vi "Go.vi"(9 "Timing Data":T1(array[cluster]), 10 "Control In":T2={"I-O.lvclass"=refnum, "Gantry"=refnum, "Dispenser"="COM1"}, 11 "Sensor Dispense in":refnum<class "Sensor Dispense.lvclass">) -> (2 "Control Out":T2={"I-O.lvclass"=refnum, "Gantry"=refnum, "Dispenser"="COM1"}, 3 "Sensor Dispense out":refnum<class "Sensor Dispense.lvclass">)   [LabVIEW 2021, in "Sensor Dispense.lvclass"]
uses:
  Sensor Dispense.lvclass
  C:/Users/hep/Documents/UCSB-CMU-GantryCode/UCSB-Gantry-HEP-main (3)/UCSB-Gantry-HEP-main/Classes/Routine/Dispense/Dispense.lvclass
  Classes/Controller/Controllers.ctl
  Classes/Controller/I-O/I-O.lvclass
  C:/Program Files (x86)/Aerotech/A3200/LabVIEW/2010/Bin/Aerotech.A3200.dll
  Program Files (x86)/Aerotech/A3200/LabVIEW/2010/Bin/Aerotech.A3200.dll
  Sensor Dispense.lvclass/Sensor Dispense.ctl
  Classes/Controller/Motion/Motion.lvclass
  Classes/Controller/Dispenser/Dispenser.lvclass
  Classes/Controller/Motion/A3200/A3200.lvclass
  Classes/Controller/Controller.lvclass
panel:
  out "error out":errorcluster
  in  "error in (no error)":errorcluster
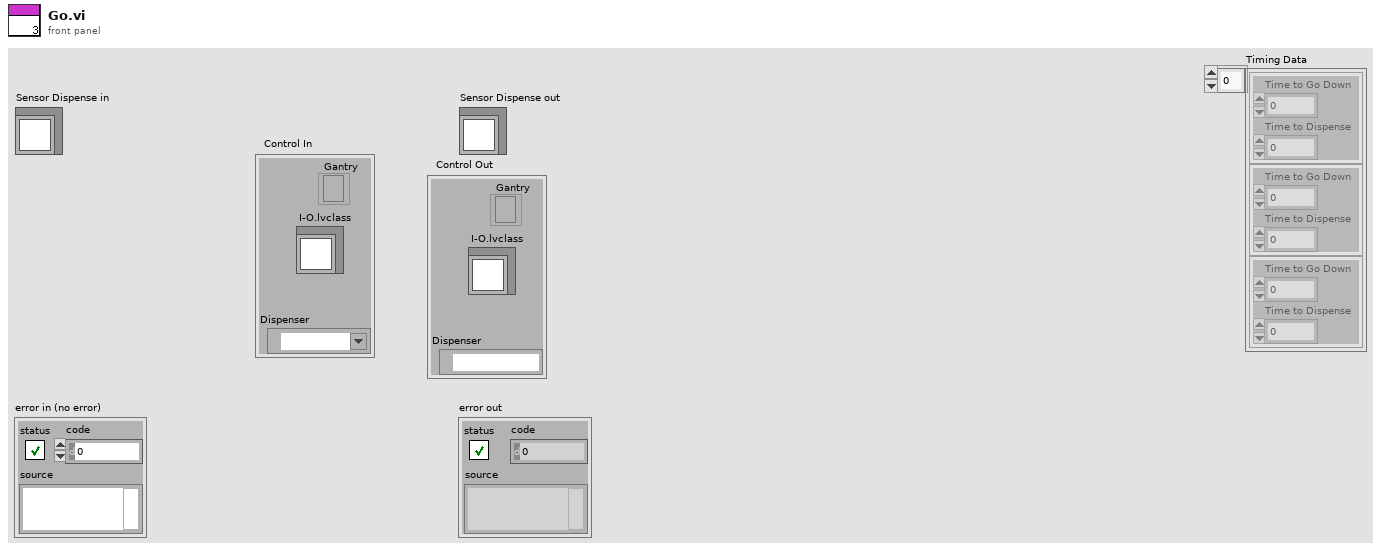
[diagram p1: front panel]
types:
  T1 = cluster{"Time to Go Down":i32, "Time to Dispense":i32}[]
  T2 = typedef "Controller.lvclass/Controllers.ctl" = cluster{"I-O.lvclass":refnum<class "I-O.lvclass">, "Gantry":refnum<k24>, "Dispenser":refnum<visa-resource-name>}
  T3 = cluster{"Endpoints":dbl[][], "Center":dbl[], "CW/CCW":dbl, "Dispense Type":enum16{"N-gon", "Square", "Arc", "Dot", "Line", "Circle"}}[]
  T4 = cluster{"Endpoints":dbl[][], "Center":dbl[], "CW/CCW":dbl, "Dispense Type":enum16{"N-gon", "Square", "Arc", "Dot", "Line", "Circle"}}
  T5 = enum16{"N-gon", "Square", "Arc", "Dot", "Line", "Circle"}
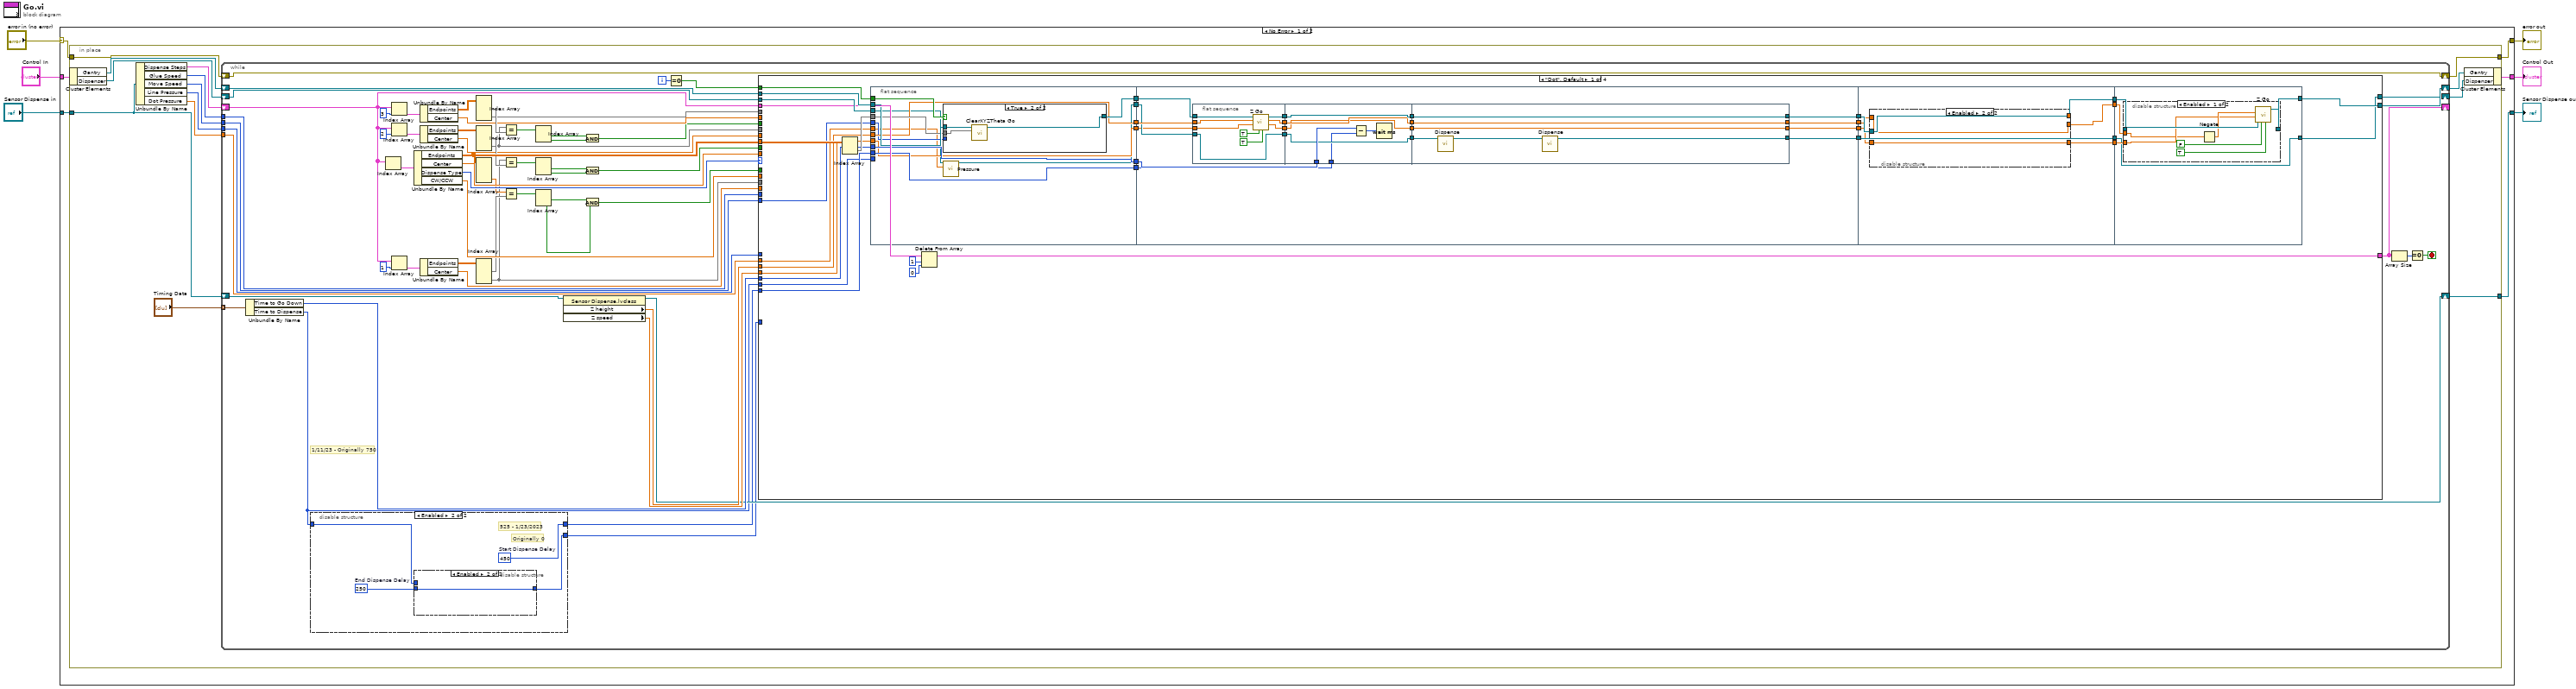
[diagram p0: block diagram]
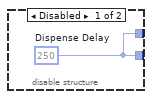
[diagram p2: hidden frame]
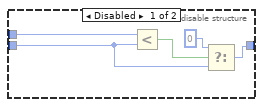
[diagram p3: hidden frame]
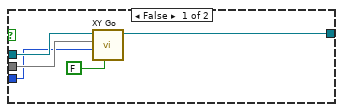
[diagram p4: hidden frame]
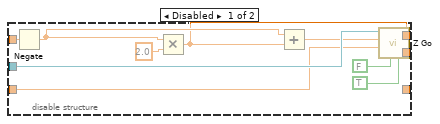
[diagram p5: hidden frame]
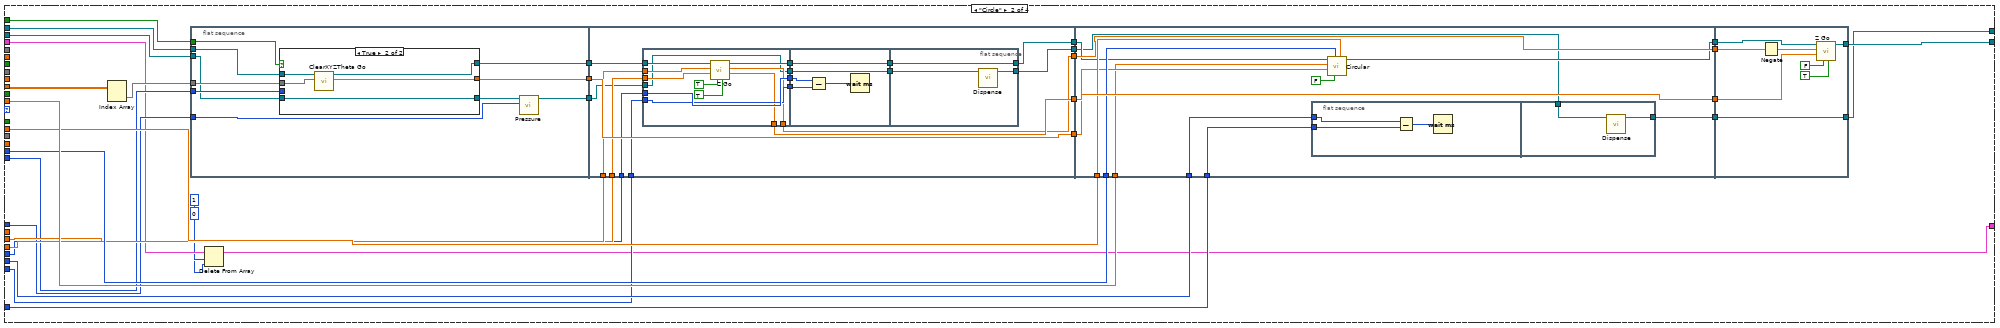
[diagram p7: hidden frame]
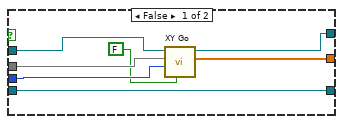
[diagram p8: hidden frame]
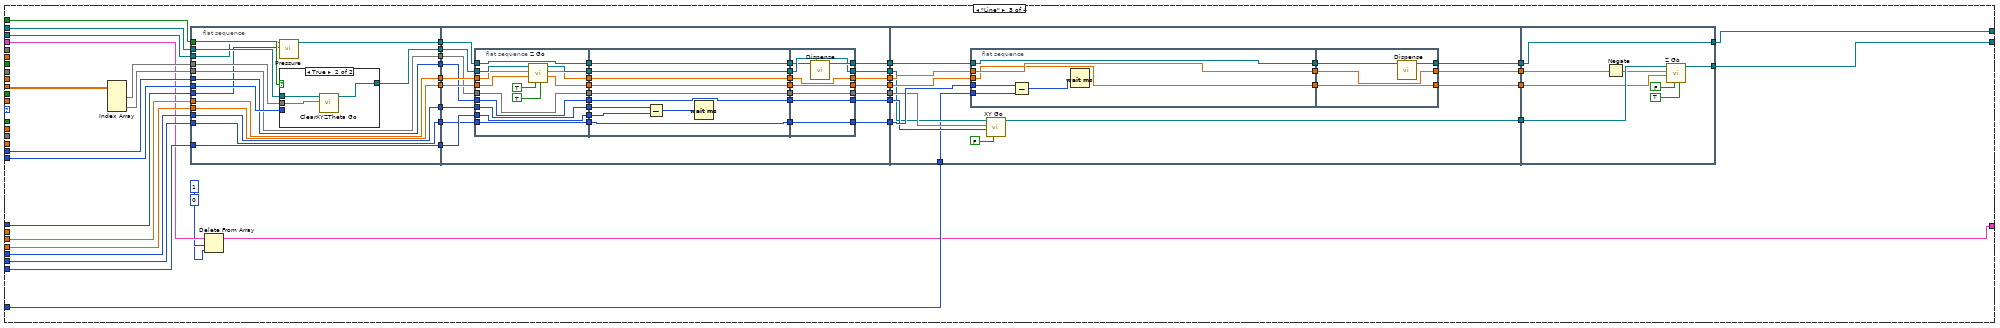
[diagram p9: hidden frame]
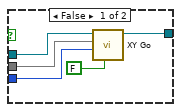
[diagram p10: hidden frame]
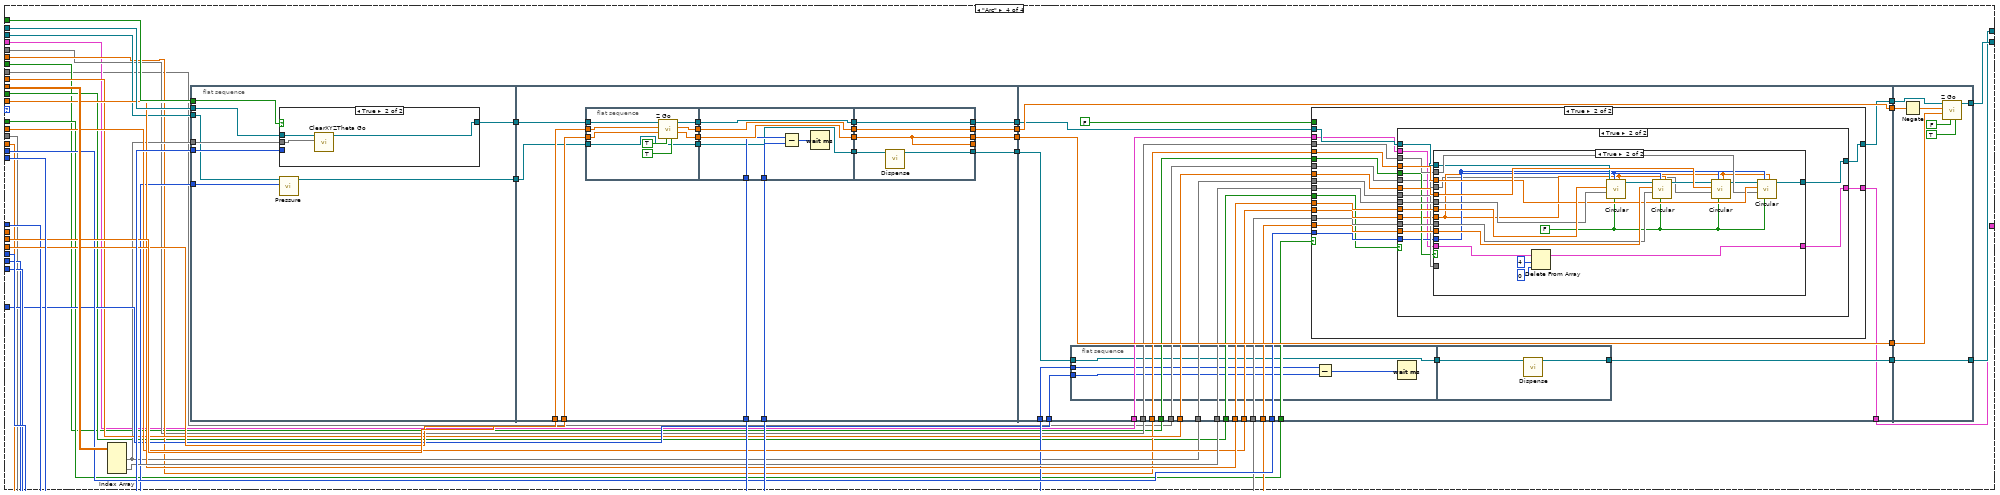
[diagram p11: hidden frame]
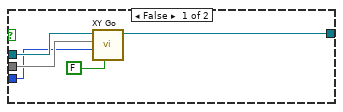
[diagram p12: hidden frame]
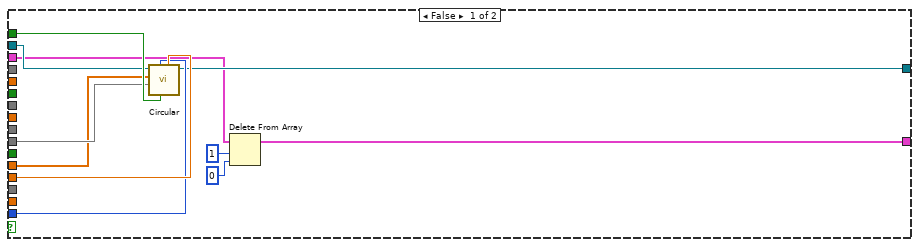
[diagram p13: hidden frame]
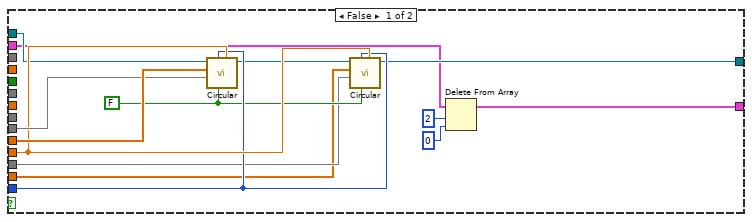
[diagram p14: hidden frame]
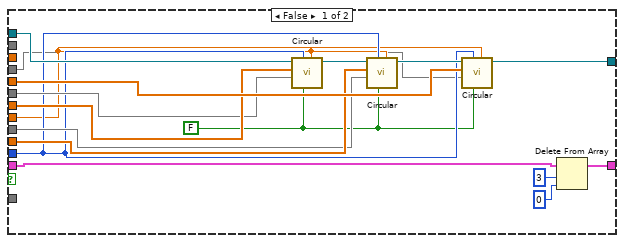
[diagram p15: hidden frame]
diagram:
  n1 = case shown="No Error" "error in (no error)" {
    selector: "error in (no error)" -> [w7 w735]
    tunnel: "Sensor Dispense in" -> [w12 w734]
    tunnel: [w11 w734] -> w5
    tunnel: "Control In" -> [w10 w733]
    tunnel: [w9 w733] -> w3
    tunnel: [w8 w735] -> w2
    frame No Error {
      n2 = in-place {
        in-place-border: w12 -> [w24]
        in-place-border: [w23] -> w11
        in-place-border: w7 -> [w17]
        in-place-border: [w16] -> w8
        n3 = in-place-cluster #1(w10) -> ("Gantry"=w25:refnum<k24>, "Dispenser"=w20:refnum<visa-resource-name>)
        n4 = Unbundle By Name(w24) -> ("Dispense Steps"=w21:T3, "Glue Speed"=w15:i32, "Move Speed"=w26:i32, "Line Pressure"=w13:i64, "Dot Pressure"=w14:dbl)
        n5 = while {
          tunnel: w26 -> [w86]
          shift-right: [w78] -> w22
          shift-left: w25 -> [w84]
          tunnel: w15 -> [w85]
          shift-right: [w70] -> w23
          shift-left: w24 -> [w82]
          shift-right: [w73] -> w18
          shift-left: w20 -> [w76]
          tunnel: "Timing Data" -> [w75] mode=indexing
          shift-right: [w66] -> w16
          shift-left: w17 -> [w66]
          tunnel: w14 -> [w68]
          tunnel: w13 -> [w67]
          shift-right: [w28] -> _
          shift-left: w21 -> [w31]
          i -> [w81]
          stop <- w30 stop-if-true
          # "1/11/23 - Originally 750"
          n6 = Unbundle By Name(w75) -> ("Time to Go Down"=w74:i32, "Time to Dispense"=w64:i32)
          n7 = disable-structure shown="Enabled" {
            disable-tunnel: [w87 w91] -> w69
            disable-tunnel: [w87 w89] -> w65
            disable-tunnel: w64 -> [_ w90]
            frame Disabled {
              w87 = 250  # Dispense Delay
            }
            frame Enabled {
              w88 = 250  # End Dispense Delay
              w91 = 450  # Start Dispense Delay
              # "525 - 1/23/2023"
              # "Originally 0"
              n8 = disable-structure shown="Enabled" {
                disable-tunnel: w90 -> [w96 _]
                disable-tunnel: [w93 w97] -> w89
                disable-tunnel: w88 -> [w92 w97]
                frame Disabled {
                  n9 = Less?(x=w96, y=w92) -> (x < y?=w95:bool)
                  n10 = Select(t=0, s=w95, f=w92) -> (s? t:f=w93:i32)
                }
                frame Enabled {
                }
              }
            }
          }
          n11 = Index Array(array=w31) -> (element=w62:T4)  [unwired: 1 in]
          n12 = Index Array(array=w31, index=3) -> (element=w58:T4)
          n13 = Index Array(array=w31, index=2) -> (element=w59:T4)
          n14 = Index Array(array=w31, index=1) -> (element=w61:T4)
          n15 = Unbundle By Name(w62) -> ("Endpoints"=w53:dbl[][], "Center"=w77:dbl[], "Dispense Type"=w79:T5, "CW/CCW"=w83:dbl)
          n16 = Unbundle By Name(w58) -> ("Endpoints"=w57:dbl[][], "Center"=w36:dbl[])
          n17 = Unbundle By Name(w59) -> ("Endpoints"=w56:dbl[][], "Center"=w37:dbl[])
          n18 = Unbundle By Name(w61) -> ("Endpoints"=w60:dbl[][], "Center"=w38:dbl[])
          n19 = Index Array(array=w57) -> (element #1=w49:dbl[], element #2=w35:dbl[])  [unwired: 4 in]
          n20 = Index Array(array=w56) -> (element #1=w50:dbl[], element #2=w27:dbl[])  [unwired: 4 in]
          n21 = Index Array(array=w53) -> (element #2=w52:dbl[])  [unwired: 4 in, 1 out]
          n22 = Index Array(array=w60) -> (element #1=w51:dbl[], element #2=w39:dbl[])  [unwired: 4 in]
          n23 = Equal?(x=w27, y=w49) -> (x = y?=w44:bool[])
          n24 = Equal?(x=w39, y=w50) -> (x = y?=w45:bool[])
          n25 = Equal?(x=w52, y=w51) -> (x = y?=w48:bool[])
          n26 = Index Array(array=w44) -> (element #1=w41:bool, element #2=w40:bool)  [unwired: 2 in]
          n27 = Index Array(array=w45) -> (element #1=w43:bool, element #2=w42:bool)  [unwired: 2 in]
          n28 = Index Array(array=w48) -> (element #1=w47:bool, element #2=w46:bool)  [unwired: 2 in]
          n29 = property on="Property Node" class="Sensor Dispense.lvclass"(reference=w82) -> (reference out=w70:refnum<class "Sensor Dispense.lvclass">, "Z height"=w72:dbl, "Z speed"=w71:dbl)  [unwired: 1 in, 1 out]
          n30 = And(x=w41, y=w40) -> (x .and. y?=w32:bool)
          n31 = And(x=w43, y=w42) -> (x .and. y?=w33:bool)
          n32 = And(x=w47, y=w46) -> (x .and. y?=w34:bool)
          n33 = Equal To 0?(x=w81) -> (x = 0?=w80:bool)
          n34 = case shown="\"Dot\", Default" w79 {
            tunnel: w77 -> [_ w252 _ w525]
            tunnel: w84 -> [w128 w253 w381 w533]
            tunnel: w86 -> [w111 w246 w380 w531]
            tunnel: [w127 w256 w377 w521] -> w78
            tunnel: w85 -> [_ w251 w367 w524]
            tunnel: w83 -> [_ w250 _ w523]
            tunnel: w71 -> [w119 w248 w364 w527]
            tunnel: w72 -> [w120 w249 w365 w528]
            tunnel: w80 -> [w129 w247 w379 w534]
            tunnel: w76 -> [w118 w230 w371 w517]
            tunnel: w74 -> [w116 w237 w369 w530]
            tunnel: w64 -> [w121 w238 w366 w522]
            tunnel: w69 -> [w122 w236 w370 w529]
            tunnel: [w126 w231 w374 w520] -> w73
            tunnel: w53 -> [w125 w235 w373 w532]
            tunnel: w68 -> [w110 _ _ _]
            tunnel: w67 -> [_ w228 w346 w516]
            tunnel: w65 -> [_ w227 w345 w515]
            tunnel: w39 -> [_ _ _ w514]
            tunnel: w38 -> [_ _ _ w513]
            tunnel: w37 -> [_ _ _ w512]
            tunnel: w36 -> [_ _ _ w510]
            tunnel: w35 -> [_ _ _ w509]
            tunnel: w34 -> [_ _ _ w508]
            tunnel: w33 -> [_ _ _ w507]
            tunnel: w32 -> [_ _ _ w506]
            tunnel: w31 -> [w102 w226 w344 w505]
            tunnel: [w99 w223 w341 w504] -> w28
            tunnel: w27 -> [_ _ _ w503]
            frame "Dot", Default {
              n35 = Index Array(array=w125) -> (element=w124:dbl[])  [unwired: 2 in]
              n36 = flat-sequence {
                tunnel: w129 -> [w141]
                tunnel: w128 -> [w140]
                tunnel: w124 -> [w139]
                tunnel: [w138] -> w123
                tunnel: w122 -> [w135]
                tunnel: w121 -> [_]
                tunnel: w120 -> [w137]
                tunnel: w119 -> [w134]
                tunnel: w118 -> [w132]
                tunnel: [w137] -> w117
                tunnel: w116 -> [w136]
                tunnel: [w136] -> w115
                tunnel: [w135] -> w114
                tunnel: [w131] -> w113
                tunnel: [w134] -> w112
                tunnel: w111 -> [w133]
                tunnel: w110 -> [w130]
                tunnel: [w167] -> w107
                tunnel: w123 -> [w166]
                tunnel: [w163] -> w106
                tunnel: w117 -> [w162]
                tunnel: w115 -> [w161]
                tunnel: w114 -> [w160]
                tunnel: w113 -> [w159]
                tunnel: w112 -> [w156]
                tunnel: [w154] -> w105
                tunnel: [w153] -> w104
                tunnel: w107 -> [w195]
                tunnel: w106 -> [w194]
                tunnel: w105 -> [w193]
                tunnel: w104 -> [w192]
                tunnel: [w196] -> w109
                tunnel: [w195] -> w108
                tunnel: [w190] -> w103
                tunnel: [w191] -> w98
                tunnel: [w210] -> w126
                tunnel: [w213] -> w127
                tunnel: w109 -> [w214]
                tunnel: w108 -> [w210]
                tunnel: w103 -> [w212]
                tunnel: w98 -> [w211]
                frame #0 {
                  n37 = case shown="True" w141 {
                    tunnel: w140 -> [w146 w149]
                    tunnel: [w145 w148] -> w138
                    tunnel: w139 -> [w144 w147]
                    tunnel: w133 -> [w143 _]
                    frame False {
                      n38 = call "XY Go.vi"("return immediately"=FALSE, "Speed"=w143, "XY In"=w144, "Gantry In"=w146) -> ("Gantry Out"=w145:refnum<k24>)  [unwired: 5 in, 2 out]
                    }
                    frame True {
                      n39 = call "ClearXYZTheta Go.vi"("XYZTheta In"=w147, "Gantry In"=w149) -> ("Gantry Out"=w148:refnum<k24>)  [unwired: 7 in, 2 out]
                    }
                  }
                  n40 = call "Pressure.vi"("Pressure"=w130, "VISA resource name"=w132) -> ("VISA resource name out"=w131:refnum<visa-resource-name>)  [unwired: 8 in, 1 out]
                }
                frame #1 {
                  n41 = flat-sequence {
                    tunnel: w166 -> [w176]
                    tunnel: [w175] -> w164
                    tunnel: w162 -> [w169]
                    tunnel: w159 -> [w173]
                    tunnel: [w173] -> w158
                    tunnel: w156 -> [w172]
                    tunnel: [w171] -> w151
                    tunnel: [w168] -> w150
                    tunnel: [w183] -> w165
                    tunnel: w164 -> [w183]
                    tunnel: w161 -> [w182]
                    tunnel: w160 -> [w178]
                    tunnel: w158 -> [w181]
                    tunnel: [w181] -> w157
                    tunnel: [w180] -> w155
                    tunnel: [w179] -> w152
                    tunnel: w151 -> [w179]
                    tunnel: w150 -> [w180]
                    tunnel: [w189] -> w167
                    tunnel: w165 -> [w188]
                    tunnel: [w188] -> w163
                    tunnel: w157 -> [w187]
                    tunnel: w155 -> [w185]
                    tunnel: [w185] -> w154
                    tunnel: [w184] -> w153
                    tunnel: w152 -> [w184]
                    frame #0 {
                      n42 = call "Z Go.vi"("Increment"=TRUE, "Return Immediately"=TRUE, "Speed In"=w172, "Position In"=w169, "Gantry In"=w176) -> ("Speed Out"=w171:dbl, "Position Out"=w168:dbl, "Gantry Out"=w175:refnum<k24>)  [unwired: 3 in, 1 out]
                    }
                    frame #1 {
                      n43 = Subtract(x=w182, y=w178) -> (x-y=w177:i32)
                      n44 = Wait (ms)(milliseconds to wait=w177) -> ()  [unwired: 1 out]
                    }
                    frame #2 {
                      n45 = call "Dispense.vi"("Dispenser In"=w187) -> ("Dispenser Out"=w186:refnum<visa-resource-name>)  [unwired: 9 in, 1 out]
                      n46 = call "Dispense.vi"("Dispenser In"=w186) -> ("Dispenser Out"=w189:refnum<visa-resource-name>)  [unwired: 9 in, 1 out]
                    }
                  }
                }
                frame #2 {
                  n47 = disable-structure shown="Enabled" {
                    disable-tunnel: [w206 w209] -> w196
                    disable-tunnel: w194 -> [w205 w209]
                    disable-tunnel: w193 -> [w204 w207]
                    disable-tunnel: w192 -> [w201 w208]
                    disable-tunnel: [w197 _] -> _
                    disable-tunnel: [_ w208] -> w191
                    disable-tunnel: [_ w207] -> w190
                    frame Disabled {
                      n48 = Negate(x=w204) -> (-x=w199:dbl)
                      n49 = Multiply(x=w199, y=2.0) -> (x*y=w197:dbl)
                      n50 = Add(x=w199, y=w197) -> (x+y=w200:dbl)
                      n51 = call "Z Go.vi"("Increment"=TRUE, "Return Immediately"=FALSE, "Speed In"=w201, "Position In"=w200, "Gantry In"=w205) -> ("Gantry Out"=w206:refnum<k24>)  [unwired: 3 in, 3 out]
                    }
                    frame Enabled {
                    }
                  }
                }
                frame #3 {
                  n52 = disable-structure shown="Enabled" {
                    disable-tunnel: w214 -> [w221 w222]
                    disable-tunnel: [w220 w222] -> w213
                    disable-tunnel: w212 -> [w215 _]
                    disable-tunnel: w211 -> [w216 _]
                    frame Enabled {
                      n53 = Negate(x=w215) -> (-x=w219:dbl)
                      n54 = call "Z Go.vi"("Increment"=TRUE, "Return Immediately"=FALSE, "Speed In"=w216, "Position In"=w219, "Gantry In"=w221) -> ("Gantry Out"=w220:refnum<k24>)  [unwired: 3 in, 3 out]
                    }
                    frame Disabled {
                    }
                  }
                }
              }
              n55 = Delete From Array(array=w102, length=1, index=0) -> (array with subset deleted=w99:T3)  [unwired: 1 out]
            }
            frame "Circle" {
              n56 = Index Array(array=w235) -> (element=w234:dbl[])  [unwired: 2 in]
              n57 = flat-sequence {
                tunnel: [w264] -> w255
                tunnel: w253 -> [w265]
                tunnel: w247 -> [w266]
                tunnel: w246 -> [w263]
                tunnel: [w262] -> w244
                tunnel: w234 -> [w261]
                tunnel: w230 -> [w260]
                tunnel: [w258] -> w229
                tunnel: w228 -> [w257]
                tunnel: w249 -> [w288]
                tunnel: w248 -> [w289]
                tunnel: [w295] -> w245
                tunnel: [w286] -> w243
                tunnel: [w287] -> w242
                tunnel: w244 -> [w295]
                tunnel: w255 -> [w285]
                tunnel: [w294] -> w239
                tunnel: w237 -> [w293]
                tunnel: w236 -> [w292]
                tunnel: [w282] -> w233
                tunnel: w229 -> [w281]
                tunnel: [w317] -> w254
                tunnel: [w327] -> w241
                tunnel: [w326] -> w240
                tunnel: w238 -> [w325]
                tunnel: w239 -> [w315]
                tunnel: w245 -> [w320]
                tunnel: w243 -> [w327]
                tunnel: w242 -> [w326]
                tunnel: w250 -> [w323]
                tunnel: w251 -> [w321]
                tunnel: w252 -> [w319]
                tunnel: w233 -> [w318]
                tunnel: [w324] -> w232
                tunnel: w227 -> [w316]
                tunnel: [w338] -> w256
                tunnel: w254 -> [w339]
                tunnel: w241 -> [w340]
                tunnel: w240 -> [w337]
                tunnel: w232 -> [w336]
                tunnel: [w336] -> w231
                frame #0 {
                  n58 = case shown="True" w266 {
                    tunnel: w265 -> [w273 w278]
                    tunnel: [w272 w277] -> w264
                    tunnel: w263 -> [w271 _]
                    tunnel: [w270 w275] -> w262
                    tunnel: w261 -> [w269 w276]
                    tunnel: w260 -> [w268 w274]
                    tunnel: [w268 w274] -> w259
                    frame False {
                      n59 = call "XY Go.vi"("return immediately"=FALSE, "Speed"=w271, "XY In"=w269, "Gantry In"=w273) -> ("XY Out"=w270:dbl[], "Gantry Out"=w272:refnum<k24>)  [unwired: 5 in, 1 out]
                    }
                    frame True {
                      n60 = call "ClearXYZTheta Go.vi"("XYZTheta In"=w276, "Gantry In"=w278) -> ("XYZTheta Out"=w275:dbl[], "Gantry Out"=w277:refnum<k24>)  [unwired: 7 in, 1 out]
                    }
                  }
                  n61 = call "Pressure.vi"("Pressure"=w257, "VISA resource name"=w259) -> ("VISA resource name out"=w258:refnum<visa-resource-name>)  [unwired: 8 in, 1 out]
                }
                frame #1 {
                  n62 = flat-sequence {
                    tunnel: w292 -> [w305]
                    tunnel: w293 -> [w306]
                    tunnel: [w306] -> w291
                    tunnel: [w305] -> w290
                    tunnel: w289 -> [w304]
                    tunnel: w288 -> [w303]
                    tunnel: [w302] -> w287
                    tunnel: [w301] -> w286
                    tunnel: w285 -> [w300]
                    tunnel: [w299] -> w284
                    tunnel: w281 -> [w297]
                    tunnel: [w297] -> w280
                    tunnel: w291 -> [w311]
                    tunnel: w290 -> [w310]
                    tunnel: w284 -> [w309]
                    tunnel: [w309] -> w283
                    tunnel: w280 -> [w308]
                    tunnel: [w308] -> w279
                    tunnel: [w314] -> w294
                    tunnel: w283 -> [w313]
                    tunnel: [w313] -> w282
                    tunnel: w279 -> [w312]
                    frame #0 {
                      n63 = call "Z Go.vi"("Increment"=TRUE, "Return Immediately"=TRUE ("return immediately"), "Speed In"=w304, "Position In"=w303, "Gantry In"=w300) -> ("Speed Out"=w302:dbl, "Position Out"=w301:dbl, "Gantry Out"=w299:refnum<k24>)  [unwired: 3 in, 1 out]
                    }
                    frame #1 {
                      n64 = Subtract(x=w311, y=w310) -> (x-y=w307:i32)
                      n65 = Wait (ms)(milliseconds to wait=w307) -> ()  [unwired: 1 out]
                    }
                    frame #2 {
                      n66 = call "Dispense.vi"("Dispenser In"=w312) -> ("Dispenser Out"=w314:refnum<visa-resource-name>)  [unwired: 9 in, 1 out]
                    }
                  }
                }
                frame #2 {
                  n67 = flat-sequence {
                    tunnel: w325 -> [w330]
                    tunnel: w316 -> [w328]
                    tunnel: [w332] -> w324
                    tunnel: w315 -> [w331]
                    frame #0 {
                      n68 = Subtract(x=w330, y=w328) -> (x-y=w329:i32)
                      n69 = Wait (ms)(milliseconds to wait=w329) -> ()  [unwired: 1 out]
                    }
                    frame #1 {
                      n70 = call "Dispense.vi"("Dispenser In"=w331) -> ("Dispenser Out"=w332:refnum<visa-resource-name>)  [unwired: 9 in, 1 out]
                    }
                  }
                  n71 = call "Circular.vi"("Direction"=w323, "return immediately"=FALSE, "Speed"=w321, "XY End"=w320, "XY Center"=w319, "Gantry In"=w318) -> ("Gantry Out"=w317:refnum<k24>)  [unwired: 4 in, 1 out]
                }
                frame #3 {
                  n72 = Negate(x=w340) -> (-x=w335:dbl)
                  n73 = call "Z Go.vi"("Increment"=TRUE, "Return Immediately"=FALSE, "Speed In"=w337, "Position In"=w335, "Gantry In"=w339) -> ("Gantry Out"=w338:refnum<k24>)  [unwired: 3 in, 3 out]
                }
              }
              n74 = Delete From Array(array=w226, length=1, index=0) -> (array with subset deleted=w223:T3)  [unwired: 1 out]
            }
            frame "Line" {
              n75 = Index Array(array=w373) -> (element #1=w372:dbl[], element #2=w368:dbl[])  [unwired: 4 in]
              n76 = flat-sequence {
                tunnel: w381 -> [w396]
                tunnel: w380 -> [w395]
                tunnel: w379 -> [w394]
                tunnel: [w393] -> w378
                tunnel: w372 -> [w392]
                tunnel: w371 -> [w384]
                tunnel: w370 -> [w388]
                tunnel: w369 -> [w389]
                tunnel: w368 -> [w387]
                tunnel: w367 -> [w386]
                tunnel: w366 -> [w385]
                tunnel: w365 -> [w391]
                tunnel: w364 -> [w390]
                tunnel: [w391] -> w363
                tunnel: [w390] -> w362
                tunnel: [w389] -> w360
                tunnel: [w388] -> w359
                tunnel: [w383] -> w358
                tunnel: [w387] -> w356
                tunnel: [w386] -> w354
                tunnel: [w385] -> w352
                tunnel: w346 -> [w382]
                tunnel: w378 -> [w435]
                tunnel: [w436] -> w376
                tunnel: w363 -> [w434]
                tunnel: w362 -> [w433]
                tunnel: [w430] -> w361
                tunnel: w360 -> [w428]
                tunnel: w359 -> [w426]
                tunnel: w358 -> [w423]
                tunnel: [w422] -> w357
                tunnel: w356 -> [w419]
                tunnel: [w418] -> w355
                tunnel: w354 -> [w415]
                tunnel: [w411] -> w353
                tunnel: w352 -> [w412]
                tunnel: [w410] -> w349
                tunnel: [w407] -> w347
                tunnel: w376 -> [w482]
                tunnel: [w484] -> w375
                tunnel: w361 -> [w471]
                tunnel: w357 -> [w472]
                tunnel: w355 -> [w473]
                tunnel: w353 -> [w481]
                tunnel: [w470] -> w351
                tunnel: [w480] -> w350
                tunnel: w349 -> [w478]
                tunnel: [w477] -> w348
                tunnel: w347 -> [w475]
                tunnel: w345 -> [w469]
                tunnel: [w502] -> w377
                tunnel: w375 -> [w501]
                tunnel: [w501] -> w374
                tunnel: w351 -> [w500]
                tunnel: w350 -> [w499]
                tunnel: w348 -> [w497]
                frame #0 {
                  n77 = call "Pressure.vi"("Pressure"=w382, "VISA resource name"=w384) -> ("VISA resource name out"=w383:refnum<visa-resource-name>)  [unwired: 8 in, 1 out]
                  n78 = case shown="True" w394 {
                    tunnel: w396 -> [w401 w404]
                    tunnel: w395 -> [w400 _]
                    tunnel: [w399 w403] -> w393
                    tunnel: w392 -> [w398 w402]
                    frame False {
                      n79 = call "XY Go.vi"("return immediately"=FALSE, "Speed"=w400, "XY In"=w398, "Gantry In"=w401) -> ("Gantry Out"=w399:refnum<k24>)  [unwired: 5 in, 2 out]
                    }
                    frame True {
                      n80 = call "ClearXYZTheta Go.vi"("XYZTheta In"=w402, "Gantry In"=w404) -> ("Gantry Out"=w403:refnum<k24>)  [unwired: 7 in, 2 out]
                    }
                  }
                }
                frame #1 {
                  n81 = flat-sequence {
                    tunnel: w435 -> [w450]
                    tunnel: w434 -> [w449]
                    tunnel: w433 -> [w448]
                    tunnel: [w446] -> w432
                    tunnel: [w445] -> w429
                    tunnel: w428 -> [w445]
                    tunnel: [w444] -> w427
                    tunnel: w426 -> [w444]
                    tunnel: [w443] -> w424
                    tunnel: w423 -> [w443]
                    tunnel: [w442] -> w420
                    tunnel: w419 -> [w442]
                    tunnel: [w441] -> w416
                    tunnel: w415 -> [w441]
                    tunnel: [w440] -> w413
                    tunnel: w412 -> [w440]
                    tunnel: [w439] -> w408
                    tunnel: [w438] -> w405
                    tunnel: w432 -> [w460]
                    tunnel: [w460] -> w431
                    tunnel: w429 -> [w459]
                    tunnel: w427 -> [w454]
                    tunnel: [w458] -> w425
                    tunnel: w424 -> [w458]
                    tunnel: [w457] -> w421
                    tunnel: w420 -> [w457]
                    tunnel: [w456] -> w417
                    tunnel: w416 -> [w456]
                    tunnel: [w455] -> w414
                    tunnel: w413 -> [w455]
                    tunnel: [w453] -> w409
                    tunnel: w408 -> [w453]
                    tunnel: [w452] -> w406
                    tunnel: w405 -> [w452]
                    tunnel: [w468] -> w436
                    tunnel: w431 -> [w467]
                    tunnel: [w467] -> w430
                    tunnel: w425 -> [w463]
                    tunnel: [w466] -> w422
                    tunnel: w421 -> [w466]
                    tunnel: [w465] -> w418
                    tunnel: w417 -> [w465]
                    tunnel: w414 -> [w464]
                    tunnel: [w464] -> w411
                    tunnel: [w462] -> w410
                    tunnel: w409 -> [w462]
                    tunnel: [w461] -> w407
                    tunnel: w406 -> [w461]
                    frame #0 {
                      n82 = call "Z Go.vi"("Increment"=TRUE, "Return Immediately"=TRUE, "Speed In"=w448, "Position In"=w449, "Gantry In"=w450) -> ("Speed Out"=w438:dbl, "Position Out"=w439:dbl, "Gantry Out"=w446:refnum<k24>)  [unwired: 3 in, 1 out]
                    }
                    frame #1 {
                      n83 = Subtract(x=w459, y=w454) -> (x-y=w451:i32)
                      n84 = Wait (ms)(milliseconds to wait=w451) -> ()  [unwired: 1 out]
                    }
                    frame #2 {
                      n85 = call "Dispense.vi"("Dispenser In"=w463) -> ("Dispenser Out"=w468:refnum<visa-resource-name>)  [unwired: 9 in, 1 out]
                    }
                  }
                }
                frame #2 {
                  n86 = flat-sequence {
                    tunnel: [w490] -> w483
                    tunnel: [w488] -> w479
                    tunnel: [w487] -> w476
                    tunnel: w482 -> [w490]
                    tunnel: w481 -> [w489]
                    tunnel: w478 -> [w488]
                    tunnel: w475 -> [w487]
                    tunnel: w469 -> [w485]
                    tunnel: [w494] -> w484
                    tunnel: w483 -> [w493]
                    tunnel: [w492] -> w480
                    tunnel: w479 -> [w492]
                    tunnel: [w491] -> w477
                    tunnel: w476 -> [w491]
                    frame #0 {
                      n87 = Subtract(x=w489, y=w485) -> (x-y=w486:i32)
                      n88 = Wait (ms)(milliseconds to wait=w486) -> ()  [unwired: 1 out]
                    }
                    frame #1 {
                      n89 = call "Dispense.vi"("Dispenser In"=w493) -> ("Dispenser Out"=w494:refnum<visa-resource-name>)  [unwired: 9 in, 1 out]
                    }
                  }
                  n90 = call "XY Go.vi"("return immediately"=FALSE, "Speed"=w473, "XY In"=w472, "Gantry In"=w471) -> ("Gantry Out"=w470:refnum<k24>)  [unwired: 5 in, 2 out]
                }
                frame #3 {
                  n91 = Negate(x=w499) -> (-x=w498:dbl)
                  n92 = call "Z Go.vi"("Increment"=TRUE, "Return Immediately"=FALSE, "Speed In"=w497, "Position In"=w498, "Gantry In"=w500) -> ("Gantry Out"=w502:refnum<k24>)  [unwired: 3 in, 3 out]
                }
              }
              n93 = Delete From Array(array=w344, length=1, index=0) -> (array with subset deleted=w341:T3)  [unwired: 1 out]
            }
            frame "Arc" {
              n94 = Index Array(array=w532) -> (element #1=w511:dbl[], element #2=w526:dbl[])  [unwired: 4 in]
              n95 = flat-sequence {
                tunnel: [w550] -> w542
                tunnel: w534 -> [w549]
                tunnel: w533 -> [w548]
                tunnel: w511 -> [w547]
                tunnel: w531 -> [w546]
                tunnel: [w545] -> w518
                tunnel: w517 -> [w544]
                tunnel: w516 -> [w543]
                tunnel: w542 -> [w575]
                tunnel: [w576] -> w541
                tunnel: [w572] -> w540
                tunnel: [w569] -> w539
                tunnel: [w566] -> w538
                tunnel: w530 -> [w565]
                tunnel: w529 -> [w564]
                tunnel: w528 -> [w563]
                tunnel: w527 -> [w562]
                tunnel: w518 -> [w561]
                tunnel: w541 -> [w619]
                tunnel: [w620] -> w537
                tunnel: w540 -> [w610]
                tunnel: w539 -> [w623]
                tunnel: [w623] -> w536
                tunnel: w538 -> [w622]
                tunnel: [w622] -> w535
                tunnel: w526 -> [w613]
                tunnel: w525 -> [w612]
                tunnel: w524 -> [w614]
                tunnel: w523 -> [w616]
                tunnel: w522 -> [w621]
                tunnel: [w611] -> w519
                tunnel: w515 -> [w617]
                tunnel: w514 -> [w609]
                tunnel: w513 -> [w608]
                tunnel: w512 -> [w607]
                tunnel: w511 -> [w606]
                tunnel: w510 -> [w605]
                tunnel: w509 -> [w604]
                tunnel: w508 -> [w603]
                tunnel: w507 -> [w602]
                tunnel: w506 -> [w601]
                tunnel: w505 -> [w600]
                tunnel: [w599] -> w504
                tunnel: w503 -> [w598]
                tunnel: [w732] -> w521
                tunnel: w537 -> [w731]
                tunnel: [w731] -> w520
                tunnel: w536 -> [w729]
                tunnel: w535 -> [w727]
                tunnel: w519 -> [w730]
                frame #0 {
                  n96 = case shown="True" w549 {
                    tunnel: [w555 w558] -> w550
                    tunnel: w548 -> [w554 w557]
                    tunnel: w547 -> [w553 w556]
                    tunnel: w546 -> [w552 _]
                    frame False {
                      n97 = call "XY Go.vi"("return immediately"=FALSE, "Speed"=w552, "XY In"=w553, "Gantry In"=w554) -> ("Gantry Out"=w555:refnum<k24>)  [unwired: 5 in, 2 out]
                    }
                    frame True {
                      n98 = call "ClearXYZTheta Go.vi"("XYZTheta In"=w556, "Gantry In"=w557) -> ("Gantry Out"=w558:refnum<k24>)  [unwired: 7 in, 2 out]
                    }
                  }
                  n99 = call "Pressure.vi"("Pressure"=w543, "VISA resource name"=w544) -> ("VISA resource name out"=w545:refnum<visa-resource-name>)  [unwired: 8 in, 1 out]
                }
                frame #1 {
                  n100 = flat-sequence {
                    tunnel: w575 -> [w585]
                    tunnel: [w583] -> w574
                    tunnel: [w582] -> w571
                    tunnel: [w581] -> w570
                    tunnel: w563 -> [w580]
                    tunnel: w562 -> [w579]
                    tunnel: w561 -> [w577]
                    tunnel: [w577] -> w560
                    tunnel: w574 -> [w592]
                    tunnel: [w592] -> w573
                    tunnel: w571 -> [w591]
                    tunnel: w570 -> [w590]
                    tunnel: [w591] -> w568
                    tunnel: [w590] -> w567
                    tunnel: w565 -> [w589]
                    tunnel: w564 -> [w588]
                    tunnel: w560 -> [w587]
                    tunnel: [w587] -> w559
                    tunnel: [w597] -> w576
                    tunnel: w573 -> [w596]
                    tunnel: [w596] -> w572
                    tunnel: [w595] -> w569
                    tunnel: w568 -> [w595]
                    tunnel: w567 -> [w594]
                    tunnel: [w594] -> _
                    tunnel: [w594] -> w566
                    tunnel: w559 -> [w593]
                    frame #0 {
                      n101 = call "Z Go.vi"("Increment"=TRUE, "Return Immediately"=TRUE, "Speed In"=w579, "Position In"=w580, "Gantry In"=w585) -> ("Speed Out"=w581:dbl, "Position Out"=w582:dbl, "Gantry Out"=w583:refnum<k24>)  [unwired: 3 in, 1 out]
                    }
                    frame #1 {
                      n102 = Subtract(x=w589, y=w588) -> (x-y=w586:i32)
                      n103 = Wait (ms)(milliseconds to wait=w586) -> ()  [unwired: 1 out]
                    }
                    frame #2 {
                      n104 = call "Dispense.vi"("Dispenser In"=w593) -> ("Dispenser Out"=w597:refnum<visa-resource-name>)  [unwired: 9 in, 1 out]
                    }
                  }
                }
                frame #2 {
                  n105 = flat-sequence {
                    tunnel: [w720] -> w618
                    tunnel: w621 -> [w722]
                    tunnel: w619 -> [w720]
                    tunnel: w617 -> [w719]
                    tunnel: [w724] -> w620
                    tunnel: w618 -> [w723]
                    frame #0 {
                      n106 = Subtract(x=w722, y=w719) -> (x-y=w721:i32)
                      n107 = Wait (ms)(milliseconds to wait=w721) -> ()  [unwired: 1 out]
                    }
                    frame #1 {
                      n108 = call "Dispense.vi"("Dispenser In"=w723) -> ("Dispenser Out"=w724:refnum<visa-resource-name>)  [unwired: 9 in, 1 out]
                    }
                  }
                  n109 = case shown="True" w603 {
                    tunnel: w616 -> [w634 w649]
                    tunnel: FALSE ("return immediately") -> [w633 _]
                    tunnel: w614 -> [w632 w648]
                    tunnel: w613 -> [w631 w650]
                    tunnel: w612 -> [w630 w651]
                    tunnel: [w629 w638] -> w611
                    tunnel: w610 -> [w628 w639]
                    tunnel: w609 -> [_ w647]
                    tunnel: w608 -> [_ w646]
                    tunnel: w607 -> [_ w645]
                    tunnel: w606 -> [_ w644]
                    tunnel: w605 -> [_ w643]
                    tunnel: w604 -> [_ w642]
                    tunnel: w602 -> [_ w641]
                    tunnel: w601 -> [_ w640]
                    tunnel: w600 -> [w627 w637]
                    tunnel: [w624 w636] -> w599
                    tunnel: w598 -> [_ w635]
                    frame False {
                      n110 = call "Circular.vi"("Direction"=w634, "return immediately"=w633, "Speed"=w632, "XY End"=w631, "XY Center"=w630, "Gantry In"=w628) -> ("Gantry Out"=w629:refnum<k24>)  [unwired: 4 in, 1 out]
                      n111 = Delete From Array(array=w627, length=1, index=0) -> (array with subset deleted=w624:T3)  [unwired: 1 out]
                    }
                    frame True {
                      n112 = case shown="True" w641 {
                        tunnel: w651 -> [w665 w679]
                        tunnel: w650 -> [w664 w678]
                        tunnel: w649 -> [w663 w669]
                        tunnel: w648 -> [w662 w670]
                        tunnel: w647 -> [w660 w680]
                        tunnel: w646 -> [w659 w681]
                        tunnel: w645 -> [_ w677]
                        tunnel: w644 -> [_ w676]
                        tunnel: w643 -> [_ w675]
                        tunnel: w642 -> [_ w674]
                        tunnel: w640 -> [_ w673]
                        tunnel: w639 -> [w658 w672]
                        tunnel: [w656 w671] -> w638
                        tunnel: w637 -> [w655 w668]
                        tunnel: [w654 w667] -> w636
                        tunnel: w635 -> [_ w666]
                        frame False {
                          w661 = FALSE
                          n113 = call "Circular.vi"("Direction"=w663, "return immediately"=w661, "Speed"=w662, "XY End"=w664, "XY Center"=w665, "Gantry In"=w658) -> ("Gantry Out"=w657:refnum<k24>)  [unwired: 4 in, 1 out]
                          n114 = call "Circular.vi"("Direction"=w663, "return immediately"=w661, "Speed"=w662, "XY End"=w660, "XY Center"=w659, "Gantry In"=w657) -> ("Gantry Out"=w656:refnum<k24>)  [unwired: 4 in, 1 out]
                          n115 = Delete From Array(array=w655, length=2, index=0) -> (array with subset deleted=w654:T3)  [unwired: 1 out]
                        }
                        frame True {
                          n116 = case shown="True" w673 {
                            tunnel: w681 -> [w697 w718]
                            tunnel: w680 -> [w694 w717]
                            tunnel: w679 -> [w696 w716]
                            tunnel: w678 -> [w695 w715]
                            tunnel: w677 -> [w698 w714]
                            tunnel: w676 -> [_ _]
                            tunnel: w675 -> [_ w713]
                            tunnel: w674 -> [_ w712]
                            tunnel: w672 -> [w693 w711]
                            tunnel: [w690 w707] -> w671
                            tunnel: w670 -> [w689 w706]
                            tunnel: w669 -> [w688 w705]
                            tunnel: w668 -> [w686 w703]
                            tunnel: [w685 w702] -> w667
                            tunnel: w666 -> [w682 w699]
                            frame False {
                              w687 = FALSE
                              n117 = call "Circular.vi"("Direction"=w688, "return immediately"=w687, "Speed"=w689, "XY End"=w695, "XY Center"=w696, "Gantry In"=w693) -> ("Gantry Out"=w692:refnum<k24>)  [unwired: 4 in, 1 out]
                              n118 = call "Circular.vi"("Direction"=w688, "return immediately"=w687, "Speed"=w689, "XY End"=w694, "XY Center"=w697, "Gantry In"=w692) -> ("Gantry Out"=w691:refnum<k24>)  [unwired: 4 in, 1 out]
                              n119 = call "Circular.vi"("Direction"=w688, "return immediately"=w687, "Speed"=w689, "XY End"=w682, "XY Center"=w698, "Gantry In"=w691) -> ("Gantry Out"=w690:refnum<k24>)  [unwired: 4 in, 1 out]
                              n120 = Delete From Array(array=w686, length=3, index=0) -> (array with subset deleted=w685:T3)  [unwired: 1 out]
                            }
                            frame True {
                              w704 = FALSE
                              n121 = Delete From Array(array=w703, length=4, index=0) -> (array with subset deleted=w702:T3)  [unwired: 1 out]
                              n122 = call "Circular.vi"("Direction"=w705, "return immediately"=w704, "Speed"=w706, "XY End"=w715, "XY Center"=w716, "Gantry In"=w711) -> ("Gantry Out"=w710:refnum<k24>)  [unwired: 4 in, 1 out]
                              n123 = call "Circular.vi"("Direction"=w705, "return immediately"=w704, "Speed"=w706, "XY End"=w717, "XY Center"=w718, "Gantry In"=w710) -> ("Gantry Out"=w709:refnum<k24>)  [unwired: 4 in, 1 out]
                              n124 = call "Circular.vi"("Direction"=w705, "return immediately"=w704, "Speed"=w706, "XY End"=w699, "XY Center"=w714, "Gantry In"=w709) -> ("Gantry Out"=w708:refnum<k24>)  [unwired: 4 in, 1 out]
                              n125 = call "Circular.vi"("Direction"=w705, "return immediately"=w704, "Speed"=w706, "XY End"=w712, "XY Center"=w713, "Gantry In"=w708) -> ("Gantry Out"=w707:refnum<k24>)  [unwired: 4 in, 1 out]
                            }
                          }
                        }
                      }
                    }
                  }
                }
                frame #3 {
                  n126 = Negate(x=w729) -> (-x=w728:dbl)
                  n127 = call "Z Go.vi"("Increment"=TRUE, "Return Immediately"=FALSE, "Speed In"=w727, "Position In"=w728, "Gantry In"=w730) -> ("Gantry Out"=w732:refnum<k24>)  [unwired: 3 in, 3 out]
                }
              }
            }
          }
          n128 = Array Size(array=w28) -> (size(s)=w29:i32)
          n129 = Equal To 0?(x=w29) -> (x = 0?=w30:bool)
        }
        n130 = in-place-cluster #1("Gantry"=w22, "Dispenser"=w18) -> (w9:T2)
      }
    }
    frame Error {
    }
  }
  "error out" <- w2
  "Sensor Dispense out" <- w5
  "Control Out" <- w3
